vi "Degres2seconds.vi"(8 "Input DEC":dbl=35996.6916 caption="DEC  [°]" format="%.6f", 11 "Input RA":dbl=70342.56719999999 caption="RA  [°]" format="%.6f") -> (0 "DEC-sec":dbl=70342.56719999999 caption="DEC [hms]" format="%<%H:%M:%S%1u>t", 3 "RA-sec":dbl=70342.56719999999 caption="RA [hms]" format="%<%H:%M:%S%1u>t")   [LabVIEW 2011]
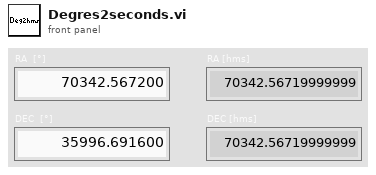
[diagram p1: front panel]
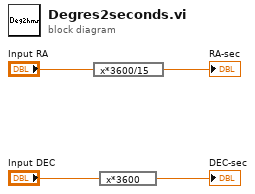
[diagram p0: block diagram]
diagram:
  n1 = expression code="x*3600/15"("Input RA") -> (→"RA-sec":dbl)
  n2 = expression code="x*3600"("Input DEC") -> (→"DEC-sec":dbl)
